vi "HDF5_Init_Noise_Refs.vi"(5 "HDF5 file ref":T1 format="%.0x", 9 "File Exists?":bool, 11 "error in":errorcluster) -> (4 "NoiseRefs":T2[](array[typedef]) {"TimeStamp_df_dset" format="%.0x"; "sum_dset" format="%.0x"; "df_dset" format="%.0x"; "TimeStamp_dset" format="%.0x"; "SumdSpectrum_dset" format="%.0x"; "TimeString_dset" format="%.0x"; "Group_ref" format="%.0x"}, 6 "HDF5 file ref":T1 format="%.0x", 15 "error out":errorcluster)   [LabVIEW 2018]
doc: "Set up the HDF5 data structure and initialize the references for the Noise1, Noise2, Noise3, and Noise4 Datasets (tables).\n\nData structure:\nNoise1 (Dataset) - 1024 element Double array (waveform) \nNoise2 (Dataset) - 1024 element Double array (waveform) \nNoise3 (Dataset) - 1024 element Double array (waveform) \nNoise4 (Dataset) - 1024 element Double array (waveform)"
uses:
  HDF5_Noise_refs.ctl
  <vilib>/addons/h5labview2/base/hid_t.ctl
  lib_path_mod_20200519.vi
  <vilib>/addons/h5labview2/base/H5Equery.vi
  <vilib>/addons/h5labview2/base/lib_path.vi
  <vilib>/addons/h5labview2/attrib/H5Awrite.llb/H5Awrite.xnode
  <vilib>/addons/h5labview2/group/H5G.lvlib
  <vilib>/addons/h5labview2/dataset/H5D.lvlib
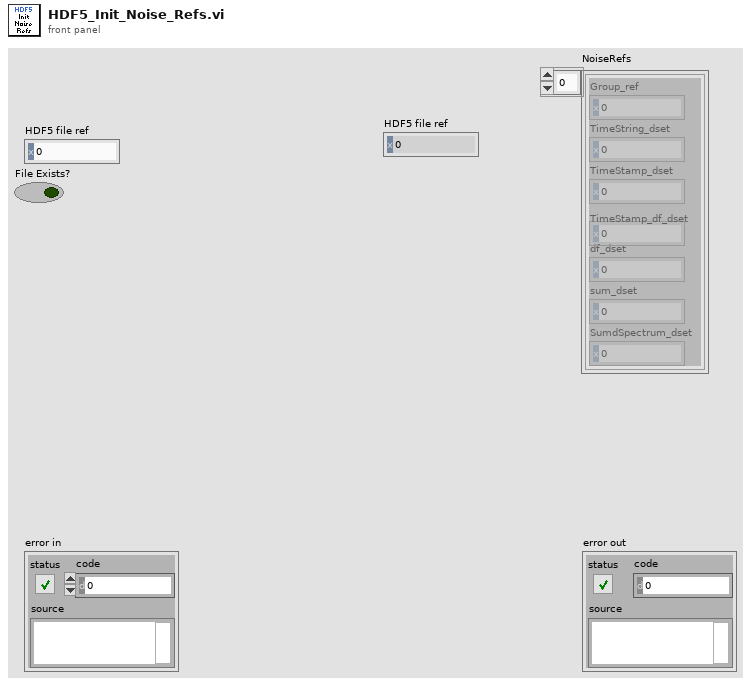
[diagram p1: front panel]
types:
  T1 = typedef "hid_t.ctl" = i32
  T2 = typedef "HDF5_Noise_refs.ctl" = cluster{"Group_ref":T1, "TimeString_dset":T1, "TimeStamp_dset":T1, "TimeStamp_df_dset":T1, "df_dset":T1, "sum_dset":T1, "SumdSpectrum_dset":T1}
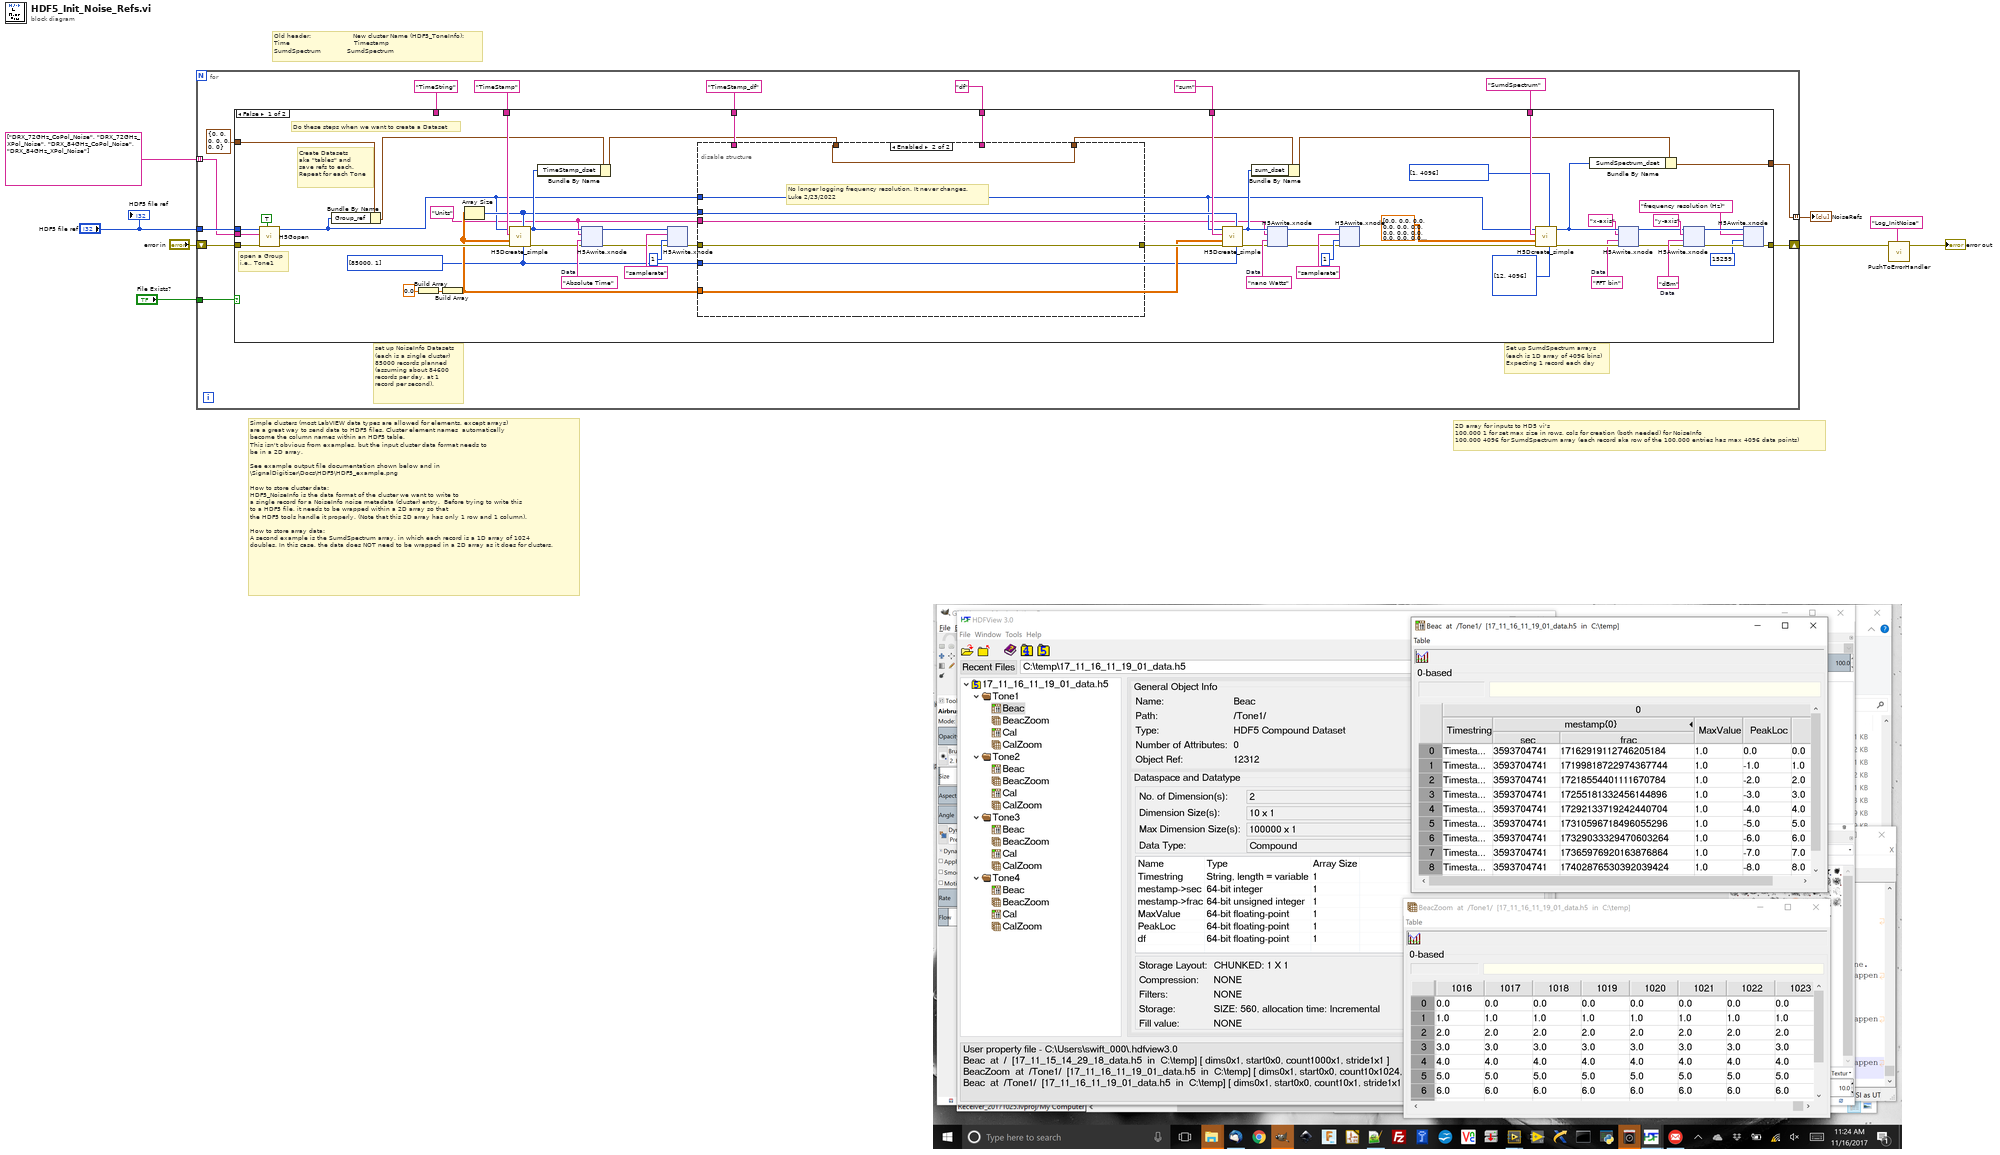
[diagram p0: block diagram]
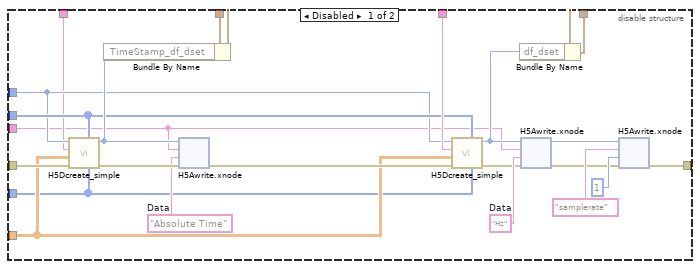
[diagram p2: hidden frame]
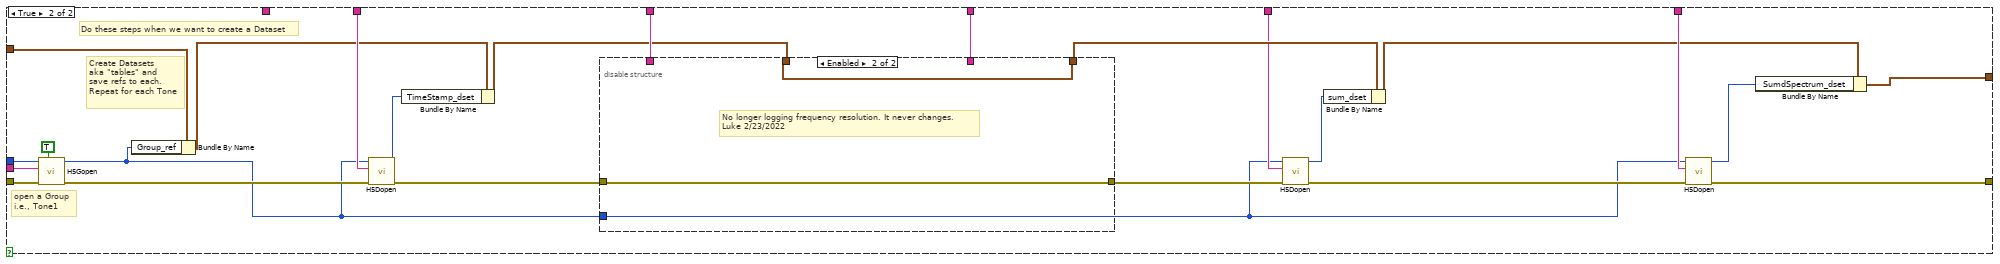
[diagram p3: hidden frame]
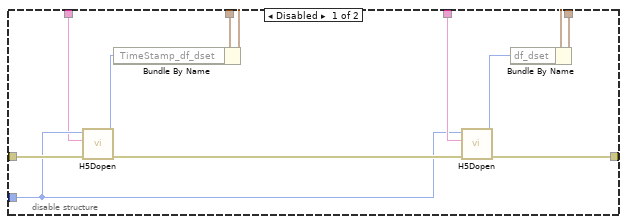
[diagram p4: hidden frame]
diagram:
  # "Simple clusters (most LabVIEW data types are allowed for elements, except arrays) \nare a great way to send data to HDF5 files. Cluster element names  automatically\nbecome the column names within an HDF5 table.\nThis isn't obvious from examples, but the input cluster data format needs to \nbe in a 2D array.\n\nSee example output file documentation shown below and in\n\\SignalDigitizer\\Docs\\HDF5\\HDF5_example.png\n\nHow to store cluster data:\nHDF5_NoiseInfo is the data format of the cluster we want to write to \na single record for a NoiseInfo noise metadata (cluster) entry.  Before trying to write this \nto a HDF5 file, it needs to be wrapped within a 2D array so that \nthe HDF5 tools handle it properly. (Note that this 2D array has only 1 row and 1 column).\n\nHow to store array data:\nA second example is the SumdSpectrum array, in which each record is a 1D array of 1024 \ndoubles. In this case, the data does NOT need to be wrapped in a 2D array as it does for clusters."
  # "2D array for inputs to HD5 vi's\n100,000 1 for set max size in rows, cols for creation (both needed) for NoiseInfo\n100,000 4096 for SumdSpectrum array (each record aka row of the 100,000 entries has max 4096 data points)"
  # "Old header:                     New cluster Name (HDF5_ToneInfo):\nTime                                Timestamp\nSumdSpectrum             SumdSpectrum"
  n1 = for {
    tunnel: "HDF5 file ref" -> [w21]
    shift-right: [w14] -> w2
    shift-left: "error in" -> [w20]
    tunnel: string[] ["DRX_72GHz_CoPol_Noise", "DRX_72GHz_XPol_Noise", "DRX_84GHz_CoPol_Noise", "DRX_84GHz_XPol_Noise"] -> [w19] mode=indexing
    tunnel: [w16] -> w8 mode=indexing
    tunnel: "File Exists?" -> [w13]
    # "Set up SumdSpectrum arrays\n(each is 1D array of 4096 bins)\nExpecting 1 record each day"
    # "set up NoiseInfo Datasets\n(each is a single cluster)\n85000 records planned\n(assuming about 84600\nrecords per day, at 1\nrecord per second)."
    n2 = case shown="False" w13 {
      tunnel: w21 -> [w77 w316]
      tunnel: w20 -> [w75 w314]
      tunnel: w19 -> [w74 w313]
      tunnel: "TimeString" ("string") -> [_ _]
      tunnel: "SumdSpectrum" ("string") -> [w73 w312]
      tunnel: [w72 w311] -> w16
      tunnel: T2 {"Group_ref"=0, "TimeString_dset"=0, "TimeStamp_dset"=0, "TimeStamp_df_dset"=0, "df_dset"=0, "sum_dset"=0, "SumdSpectrum_dset"=0} ("Cluster") -> [w71 w309]
      tunnel: [w25 w308] -> w14
      tunnel: "TimeStamp" ("string") -> [w66 w300]
      tunnel: "df" ("string") -> [w65 w299]
      tunnel: "sum" ("string") -> [w64 w298]
      tunnel: "TimeStamp_df" ("string") -> [w32 w294]
      frame False {
        w50 = "dBm"  # Data
        w54 = "FFT bin"  # Data
        w58 = "nano Watts"  # Data
        w61 = "Absolute Time"  # Data
        w27 = "Units" ("attrib name")
        w29 = u64[] [85000, 1] ("NoiseInfoArraySize")
        # "Do these steps when we want to create a Dataset"
        # "Create Datasets\naka \"tables\" and\nsave refs to each.\nRepeat for each Tone"
        # "open a Group\ni.e., Tone1"
        n3 = call <vilib>:"H5Gopen.vi"("create? (F)"=TRUE, "error in (no error)"=w75, "name"=w74, "ref in"=w77) -> ("error out"=w46:errorcluster, "group out"=w33:T1)  [unwired: 6 in]
        n4 = Bundle By Name(cluster=w71, "Group_ref"=w33) -> (w47:T2)
        n5 = Build Array(0.0 ("Timestamp")) -> (w68:dbl[])
        n6 = Build Array(w68) -> (w30:dbl[][])
        n7 = Array Size(array=w30) -> (size(s)=w34:i32[])
        n8 = call <vilib>:"H5Dcreate_simple.vi"("max size"=w29, "chunk size"=w34, "error in (no error)"=w46, "type in"=w30, "name"=w66, "ref in"=w33) -> ("error out"=w59:errorcluster, "dset out"=w60:T1)  [unwired: 4 in]
        n9 = Bundle By Name(cluster=w47, "TimeStamp_dset"=w60) -> (w28:T2)
        n10 = xnode "H5Awrite.xnode"("error in (no error)"=w59, "data"=w61, "attrib name"=w27, "ref in"=w60) -> ("error out"=w43:errorcluster, "ref out"=w42:i32)  [unwired: 3 in, 1 out]
        n11 = xnode "H5Awrite.xnode"("error in (no error)"=w43, "data"=u32 1, "attrib name"="samplerate", "ref in"=w42) -> ("error out"=w31:errorcluster)  [unwired: 3 in, 2 out]
        n12 = disable-structure shown="Enabled" {
          disable-tunnel: w65 -> [w119 _]
          disable-tunnel: [w118 w178] -> w63
          disable-tunnel: [w111 w177] -> w41
          disable-tunnel: w34 -> [w105 _]
          disable-tunnel: w33 -> [w104 _]
          disable-tunnel: w32 -> [w103 _]
          disable-tunnel: w31 -> [w102 w177]
          disable-tunnel: w30 -> [w101 _]
          disable-tunnel: w29 -> [w100 _]
          disable-tunnel: w28 -> [w99 w178]
          disable-tunnel: w27 -> [w97 _]
          frame Disabled {
            w106 = "Absolute Time"  # Data
            w117 = "Hz"  # Data
            n13 = call <vilib>:"H5Dcreate_simple.vi"("max size"=w100, "chunk size"=w105, "error in (no error)"=w102, "type in"=w101, "name"=w103, "ref in"=w104) -> ("error out"=w108:errorcluster, "dset out"=w107:T1)  [unwired: 4 in]
            n14 = Bundle By Name(cluster=w99, "TimeStamp_df_dset"=w107) -> (w98:T2)
            n15 = xnode "H5Awrite.xnode"("error in (no error)"=w108, "data"=w106, "attrib name"=w97, "ref in"=w107) -> ("error out"=w109:errorcluster)  [unwired: 3 in, 2 out]
            n16 = call <vilib>:"H5Dcreate_simple.vi"("max size"=w100, "chunk size"=w105, "error in (no error)"=w109, "type in"=w101, "name"=w119, "ref in"=w104) -> ("error out"=w115:errorcluster, "dset out"=w116:T1)  [unwired: 4 in]
            n17 = Bundle By Name(cluster=w98, "df_dset"=w116) -> (w118:T2)
            n18 = xnode "H5Awrite.xnode"("error in (no error)"=w115, "data"=w117, "attrib name"=w97, "ref in"=w116) -> ("error out"=w112:errorcluster, "ref out"=w110:i32)  [unwired: 3 in, 1 out]
            n19 = xnode "H5Awrite.xnode"("error in (no error)"=w112, "data"=u32 1, "attrib name"="samplerate", "ref in"=w110) -> ("error out"=w111:errorcluster)  [unwired: 3 in, 2 out]
          }
          frame Enabled {
            # "No longer logging frequency resolution. It never changes.\nLuke 2/23/2022"
          }
        }
        n20 = call <vilib>:"H5Dcreate_simple.vi"("max size"=w29, "chunk size"=w34, "error in (no error)"=w41, "type in"=w30, "name"=w64, "ref in"=w33) -> ("error out"=w57:errorcluster, "dset out"=w56:T1)  [unwired: 4 in]
        n21 = Bundle By Name(cluster=w63, "sum_dset"=w56) -> (w62:T2)
        n22 = xnode "H5Awrite.xnode"("error in (no error)"=w57, "data"=w58, "attrib name"=w27, "ref in"=w56) -> ("error out"=w38:errorcluster, "ref out"=w36:i32)  [unwired: 3 in, 1 out]
        n23 = xnode "H5Awrite.xnode"("error in (no error)"=w38, "data"=u32 1, "attrib name"="samplerate", "ref in"=w36) -> ("error out"=w37:errorcluster)  [unwired: 3 in, 2 out]
        n24 = call <vilib>:"H5Dcreate_simple.vi"("max size"=u64[] [12, 4096], "chunk size"=i32[] [1, 4096] ("size(s)"), "error in (no error)"=w37, "type in"=dbl[][] [[0.0, 0.0, 0.0, 0.0, 0.0, 0.0, 0.0, 0.0, 0.0, 0.0, 0.0, 0.0, 0.0, 0.0, 0.0, 0.0, 0.0, 0.0, 0.0, 0.0, 0.0, 0.0, 0.0, 0.0, 0.0, 0.0, 0.0, 0.0, 0.0, 0.0, 0.0, 0.0, 0.0, 0.0, 0.0, 0.0, 0.0, 0.0, 0.0, 0.0, 0.0, 0.0, 0.0, 0.0, 0.0, 0.0, 0.0, 0.0, 0.0, 0.0, 0.0, 0.0, 0.0, 0.0, 0.0, 0.0, 0.0, 0.0, 0.0, 0.0, 0.0, 0.0, 0.0, 0.0, 0.0, 0.0, 0.0, 0.0, 0.0, 0.0, 0.0, 0.0, 0.0, 0.0, 0.0, 0.0, 0.0, 0.0, 0.0, 0.0, 0.0, 0.0, 0.0, 0.0, 0.0, 0.0, 0.0, 0.0, 0.0, 0.0, 0.0, 0.0, 0.0, 0.0, 0.0, 0.0, 0.0, 0.0, 0.0, 0.0, 0.0, 0.0, 0.0, 0.0, 0.0, 0.0, 0.0, 0.0, 0.0, 0.0, 0.0, 0.0, 0.0, 0.0, 0.0, 0.0, 0.0, 0.0, 0.0, 0.0, 0.0, 0.0, 0.0, 0.0, 0.0, 0.0, 0.0, 0.0, 0.0, 0.0, 0.0, 0.0, 0.0, 0.0, 0.0, 0.0, 0.0, 0.0, 0.0, 0.0, 0.0, 0.0, 0.0, 0.0, 0.0, 0.0, 0.0, 0.0, 0.0, 0.0, 0.0, 0.0, 0.0, 0.0, 0.0, 0.0, 0.0, 0.0, 0.0, 0.0, 0.0, 0.0, 0.0, 0.0, 0.0, 0.0, 0.0, 0.0, 0.0, 0.0, 0.0, 0.0, 0.0, 0.0, 0.0, 0.0, 0.0, 0.0, 0.0, 0.0, 0.0, 0.0, 0.0, 0.0, 0.0, 0.0, 0.0, 0.0, 0.0, 0.0, 0.0, 0.0, 0.0, 0.0, 0.0, 0.0, 0.0, 0.0, 0.0, 0.0, 0.0, 0.0, 0.0, 0.0, 0.0, 0.0, 0.0, 0.0, 0.0, 0.0, 0.0, 0.0, 0.0, 0.0, 0.0, 0.0, 0.0, 0.0, 0.0, 0.0, 0.0, 0.0, 0.0, 0.0, 0.0, 0.0, 0.0, 0.0, 0.0, 0.0, 0.0, 0.0, 0.0, 0.0, 0.0, 0.0, 0.0, 0.0, 0.0, 0.0, 0.0, 0.0, 0.0, 0.0, 0.0, 0.0, 0.0, 0.0, 0.0, 0.0, 0.0, 0.0, 0.0, 0.0, 0.0, 0.0, 0.0, 0.0, 0.0, 0.0, 0.0, 0.0, 0.0, 0.0, 0.0, 0.0, 0.0, 0.0, 0.0, 0.0, 0.0, 0.0, 0.0, 0.0, 0.0, 0.0, 0.0, 0.0, 0.0, 0.0, 0.0, 0.0, 0.0, 0.0, 0.0, 0.0, 0.0, 0.0, 0.0, 0.0, 0.0, 0.0, 0.0, 0.0, 0.0, 0.0, 0.0, 0.0, 0.0, 0.0, 0.0, 0.0, 0.0, 0.0, 0.0, 0.0, 0.0, 0.0, 0.0, 0.0, 0.0, 0.0, 0.0, 0.0, 0.0, 0.0, 0.0, 0.0, 0.0, 0.0, 0.0, 0.0, 0.0, 0.0, 0.0, 0.0, 0.0, 0.0, 0.0, 0.0, 0.0, 0.0, 0.0, 0.0, 0.0, 0.0, 0.0, 0.0, 0.0, 0.0, 0.0, 0.0, 0.0, 0.0, 0.0, 0.0, 0.0, 0.0, 0.0, 0.0, 0.0, 0.0, 0.0, 0.0, 0.0, 0.0, 0.0, 0.0, 0.0, 0.0, 0.0, 0.0, 0.0, 0.0, 0.0, 0.0, 0.0, 0.0, 0.0, 0.0, 0.0, 0.0, 0.0, 0.0, 0.0, 0.0, 0.0, 0.0, 0.0, 0.0, 0.0, 0.0, 0.0, 0.0, 0.0, 0.0, 0.0, 0.0, 0.0, 0.0, 0.0, 0.0, 0.0, 0.0, 0.0, 0.0, 0.0, 0.0, 0.0, 0.0, 0.0, 0.0, 0.0, 0.0, 0.0, 0.0, 0.0, 0.0, 0.0, 0.0, 0.0, 0.0, 0.0, 0.0, 0.0, 0.0, 0.0, 0.0, 0.0, 0.0, 0.0, 0.0, 0.0, 0.0, 0.0, 0.0, 0.0, 0.0, 0.0, 0.0, 0.0, 0.0, 0.0, 0.0, 0.0, 0.0, 0.0, 0.0, 0.0, 0.0, 0.0, 0.0, 0.0, 0.0, 0.0, 0.0, 0.0, 0.0, 0.0, 0.0, 0.0, 0.0, 0.0, 0.0, 0.0, 0.0, 0.0, 0.0, 0.0, 0.0, 0.0, 0.0, 0.0, 0.0, 0.0, 0.0, 0.0, 0.0, 0.0, 0.0, 0.0, 0.0, 0.0, 0.0, 0.0, 0.0, 0.0, 0.0, 0.0, 0.0, 0.0, 0.0, 0.0, 0.0, 0.0, 0.0, 0.0, 0.0, 0.0, 0.0, 0.0, 0.0, 0.0, 0.0, 0.0, 0.0, 0.0, 0.0, 0.0, 0.0, 0.0, 0.0, 0.0, 0.0, 0.0, 0.0, 0.0, 0.0, 0.0, 0.0, 0.0, 0.0, 0.0, 0.0, 0.0, 0.0, 0.0, 0.0, 0.0, 0.0, 0.0, 0.0, 0.0, 0.0, 0.0, 0.0, 0.0, 0.0, 0.0, 0.0, 0.0, 0.0, 0.0, 0.0, 0.0, 0.0, 0.0, 0.0, 0.0, 0.0, 0.0, 0.0, 0.0, 0.0, 0.0, 0.0, 0.0, 0.0, 0.0, 0.0, 0.0, 0.0, 0.0, 0.0, 0.0, 0.0, 0.0, 0.0, 0.0, 0.0, 0.0, 0.0, 0.0, 0.0, 0.0, 0.0, 0.0, 0.0, 0.0, 0.0, 0.0, 0.0, 0.0, 0.0, 0.0, 0.0, 0.0, 0.0, 0.0, 0.0, 0.0, 0.0, 0.0, 0.0, 0.0, 0.0, 0.0, 0.0, 0.0, 0.0, 0.0, 0.0, 0.0, 0.0, 0.0, 0.0, 0.0, 0.0, 0.0, 0.0, 0.0, 0.0, 0.0, 0.0, 0.0, 0.0, 0.0, 0.0, 0.0, 0.0, 0.0, 0.0, 0.0, 0.0, 0.0, 0.0, 0.0, 0.0, 0.0, 0.0, 0.0, 0.0, 0.0, 0.0, 0.0, 0.0, 0.0, 0.0, 0.0, 0.0, 0.0, 0.0, 0.0, 0.0, 0.0, 0.0, 0.0, 0.0, 0.0, 0.0, 0.0, 0.0, 0.0, 0.0, 0.0, 0.0, 0.0, 0.0, 0.0, 0.0, 0.0, 0.0, 0.0, 0.0, 0.0, 0.0, 0.0, 0.0, 0.0, 0.0, 0.0, 0.0, 0.0, 0.0, 0.0, 0.0, 0.0, 0.0, 0.0, 0.0, 0.0, 0.0, 0.0, 0.0, 0.0, 0.0, 0.0, 0.0, 0.0, 0.0, 0.0, 0.0, 0.0, 0.0, 0.0, 0.0, 0.0, 0.0, 0.0, 0.0, 0.0, 0.0, 0.0, 0.0, 0.0, 0.0, 0.0, 0.0, 0.0, 0.0, 0.0, 0.0, 0.0, 0.0, 0.0, 0.0, 0.0, 0.0, 0.0, 0.0, 0.0, 0.0, 0.0, 0.0, 0.0, 0.0, 0.0, 0.0, 0.0, 0.0, 0.0, 0.0, 0.0, 0.0, 0.0, 0.0, 0.0, 0.0, 0.0, 0.0, 0.0, 0.0, 0.0, 0.0, 0.0, 0.0, 0.0, 0.0, 0.0, 0.0, 0.0, 0.0, 0.0, 0.0, 0.0, 0.0, 0.0, 0.0, 0.0, 0.0, 0.0, 0.0, 0.0, 0.0, 0.0, 0.0, 0.0, 0.0, 0.0, 0.0, 0.0, 0.0, 0.0, 0.0, 0.0, 0.0, 0.0, 0.0, 0.0, 0.0, 0.0, 0.0, 0.0, 0.0, 0.0, 0.0, 0.0, 0.0, 0.0, 0.0, 0.0, 0.0, 0.0, 0.0, 0.0, 0.0, 0.0, 0.0, 0.0, 0.0, 0.0, 0.0, 0.0, 0.0, 0.0, 0.0, 0.0, 0.0, 0.0, 0.0, 0.0, 0.0, 0.0, 0.0, 0.0, 0.0, 0.0, 0.0, 0.0, 0.0, 0.0, 0.0, 0.0, 0.0, 0.0, 0.0, 0.0, 0.0, 0.0, 0.0, 0.0, 0.0, 0.0, 0.0, 0.0, 0.0, 0.0, 0.0, 0.0, 0.0, 0.0, 0.0, 0.0, 0.0, 0.0, 0.0, 0.0, 0.0, 0.0, 0.0, 0.0, 0.0, 0.0, 0.0, 0.0, 0.0, 0.0, 0.0, 0.0, 0.0, 0.0, 0.0, 0.0, 0.0, 0.0, 0.0, 0.0, 0.0, 0.0, 0.0, 0.0, 0.0, 0.0, 0.0, 0.0, 0.0, 0.0, 0.0, 0.0, 0.0, 0.0, 0.0, 0.0, 0.0, 0.0, 0.0, 0.0, 0.0, 0.0, 0.0, 0.0, 0.0, 0.0, 0.0, 0.0, 0.0, 0.0, 0.0, 0.0, 0.0, 0.0, 0.0, 0.0, 0.0, 0.0, 0.0, 0.0, 0.0, 0.0, 0.0, 0.0, 0.0, 0.0, 0.0, 0.0, 0.0, 0.0, 0.0, 0.0, 0.0, 0.0, 0.0, 0.0, 0.0, 0.0, 0.0, 0.0, 0.0, 0.0, 0.0, 0.0, 0.0, 0.0, 0.0, 0.0, 0.0, 0.0, 0.0, 0.0, 0.0, 0.0, 0.0, 0.0, 0.0, 0.0, 0.0, 0.0, 0.0, 0.0, 0.0, 0.0, 0.0, 0.0, 0.0, 0.0, 0.0, 0.0, 0.0, 0.0, 0.0, 0.0, 0.0, 0.0, 0.0, 0.0, 0.0, 0.0, 0.0, 0.0, 0.0, 0.0, 0.0, 0.0, 0.0, 0.0, 0.0, 0.0, 0.0, 0.0, 0.0, 0.0, 0.0, 0.0, 0.0, 0.0, 0.0, 0.0, 0.0, 0.0, 0.0, 0.0, 0.0, 0.0, 0.0, 0.0, 0.0, 0.0, 0.0, 0.0, 0.0, 0.0, 0.0, 0.0, 0.0, 0.0, 0.0, 0.0, 0.0, 0.0, 0.0, 0.0, 0.0, 0.0, 0.0, 0.0, 0.0, 0.0, 0.0, 0.0, 0.0, 0.0, 0.0, 0.0, 0.0, 0.0, 0.0, 0.0, 0.0, 0.0, 0.0, 0.0, 0.0, 0.0, 0.0]] ("SumdSpectrum"), "name"=w73, "ref in"=w33) -> ("error out"=w55:errorcluster, "dset out"=w53:T1)  [unwired: 4 in]
        n25 = Bundle By Name(cluster=w62, "SumdSpectrum_dset"=w53) -> (w72:T2)
        n26 = xnode "H5Awrite.xnode"("error in (no error)"=w55, "data"=w54, "attrib name"="x-axis", "ref in"=w53) -> ("error out"=w49:errorcluster, "ref out"=w48:i32)  [unwired: 3 in, 1 out]
        n27 = xnode "H5Awrite.xnode"("error in (no error)"=w49, "data"=w50, "attrib name"="y-axis", "ref in"=w48) -> ("error out"=w26:errorcluster, "ref out"=w24:i32)  [unwired: 3 in, 1 out]
        n28 = xnode "H5Awrite.xnode"("error in (no error)"=w26, "data"=u32 15259, "attrib name"="frequency resolution (Hz)", "ref in"=w24) -> ("error out"=w25:errorcluster)  [unwired: 3 in, 2 out]
      }
      frame True {
        # "Do these steps when we want to create a Dataset"
        # "Create Datasets\naka \"tables\" and\nsave refs to each.\nRepeat for each Tone"
        # "open a Group\ni.e., Tone1"
        n29 = call <vilib>:"H5Gopen.vi"("create? (F)"=TRUE, "error in (no error)"=w314, "name"=w313, "ref in"=w316) -> ("error out"=w297:errorcluster, "group out"=w295:T1)  [unwired: 6 in]
        n30 = Bundle By Name(cluster=w309, "Group_ref"=w295) -> (w296:T2)
        n31 = call <vilib>:"H5Dopen.vi"("error in (no error)"=w297, "name"=w300, "loc in"=w295) -> ("error out"=w305:errorcluster, "dset out"=w302:T1)  [unwired: 7 in]
        n32 = Bundle By Name(cluster=w296, "TimeStamp_dset"=w302) -> (w293:T2)
        n33 = disable-structure shown="Enabled" {
          disable-tunnel: [w326 w328] -> w307
          disable-tunnel: w305 -> [w325 w327]
          disable-tunnel: [w324 w327] -> w304
          disable-tunnel: w299 -> [w322 _]
          disable-tunnel: w295 -> [w320 _]
          disable-tunnel: w294 -> [w319 _]
          disable-tunnel: w293 -> [w318 w328]
          frame Disabled {
            n34 = call <vilib>:"H5Dopen.vi"("name"=w319, "loc in"=w320) -> ("dset out"=w321:T1)  [unwired: 8 in, 1 out]
            n35 = Bundle By Name(cluster=w318, "TimeStamp_df_dset"=w321) -> (w317:T2)
            n36 = call <vilib>:"H5Dopen.vi"("error in (no error)"=w325, "name"=w322, "loc in"=w320) -> ("error out"=w324:errorcluster, "dset out"=w323:T1)  [unwired: 7 in]
            n37 = Bundle By Name(cluster=w317, "df_dset"=w323) -> (w326:T2)
          }
          frame Enabled {
            # "No longer logging frequency resolution. It never changes.\nLuke 2/23/2022"
          }
        }
        n38 = call <vilib>:"H5Dopen.vi"("error in (no error)"=w304, "name"=w298, "loc in"=w295) -> ("error out"=w303:errorcluster, "dset out"=w301:T1)  [unwired: 7 in]
        n39 = Bundle By Name(cluster=w307, "sum_dset"=w301) -> (w306:T2)
        n40 = call <vilib>:"H5Dopen.vi"("error in (no error)"=w303, "name"=w312, "loc in"=w295) -> ("error out"=w308:errorcluster, "dset out"=w310:T1)  [unwired: 7 in]
        n41 = Bundle By Name(cluster=w306, "SumdSpectrum_dset"=w310) -> (w311:T2)
      }
    }
  }
  "NoiseRefs" <- w8
  n42 = call "PushToErrorHandler.vi"("ErrorIn"=w2, "ErrorLocation"="Log_InitNoise") -> ("ErrorOut"=→"error out":errorcluster)  [unwired: 5 in]
  "HDF5 file ref" <- "HDF5 file ref"
